vi "Tx Event Init.vi"(8 "error in (no error)":errorcluster, 9 "Channel Number":u32, 10 "signal list":refnum<k21>[](array[refnum])=["CANCyclicSignal1\nnixnet_example.CAN_Cluster", "CANCyclicSignal2\nnixnet_example.CAN_Cluster", "CANCyclicSignal3\nnixnet_example.CAN_Cluster"], 11 "FPGA Refnum":T2) -> (0 "error out":errorcluster, 3 "Tx Event":T1)   [LabVIEW 2020, in "985x Support Addon Engine.lvlib"]
uses:
  985x Support Addon Engine.lvlib
  Types/FPGA Refnum.ctl
  Types/Tx Event Session.ctl
  <vilib>/xnet/xnet.llb/XNET Create Session (Conversion).vi
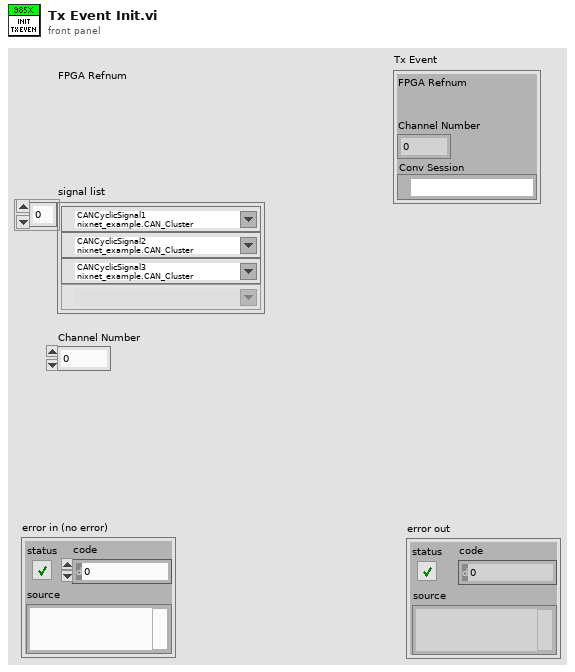
[diagram p1: front panel]
types:
  T1 = typedef "985x Support Addon Engine.lvlib/Tx Event Session.ctl" = cluster{"FPGA Refnum":T2, "Channel Number":u32, "Conv Session":refnum<k21>}
  T2 = typedef "985x Support Addon Engine.lvlib/FPGA Refnum.ctl" = refnum<k20>
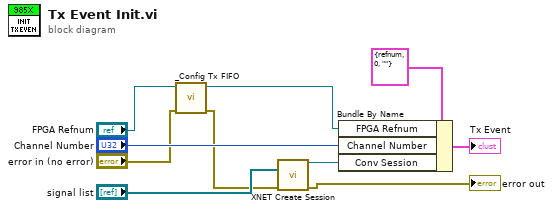
[diagram p0: block diagram]
diagram:
  n1 = call "_Config Tx FIFO.vi"("error in (no error)"="error in (no error)", "Refnum in"="FPGA Refnum") -> ("error out"=w2:errorcluster, "Refnum out"=w7:T2)  [unwired: 8 in]
  n2 = call-poly <vilib>:"XNET Create Session.vi"("signal list"="signal list", "error in (no error)"=w2) -> ("session out"=w5:refnum<k21>, "error out"=→"error out":errorcluster)  [unwired: 12 in]
  n3 = Bundle By Name(cluster=T1 {"FPGA Refnum"=refnum, "Channel Number"=0, "Conv Session"=""} ("Tx Event"), "FPGA Refnum"=w7, "Channel Number"="Channel Number", "Conv Session"=w5) -> (→"Tx Event":T1)
